vi "Can_File_be_Editted.vi"(0 "Filename":path) -> (1 "File Permissions OK?":bool, 2 "File Status":T1=enum."Directory structure cannot be created", 3 "Comment String":string="Directory structure cannot be created", 4 "Cannot create directory":path)   [LabVIEW 2016]
uses:
  File_Status.ctl
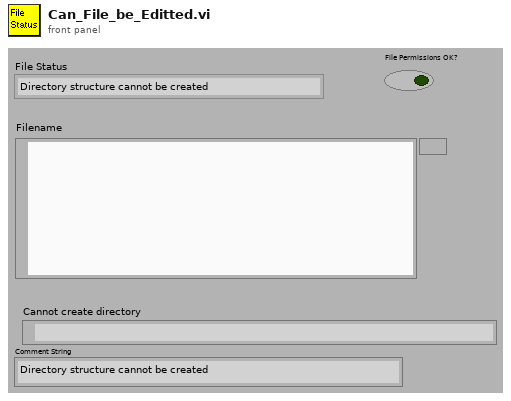
[diagram p1: front panel]
types:
  T1 = typedef "File_Status.ctl" = enum16{"Invalid Path", "File Does not Exist", "This is a folder pathname", "Generic File Error", "Directory structure cannot be created", "File cannot be created", "File can be created", "File exist but read only", "File exist but no access", "File exist with read and write access"}
  T2 = enum16{"read/write", "read-only", "write-only", "write-only (truncate)"}
  T3 = enum16{"open", "replace", "create", "open or create", "replace or create", "replace or create with confirmation"}
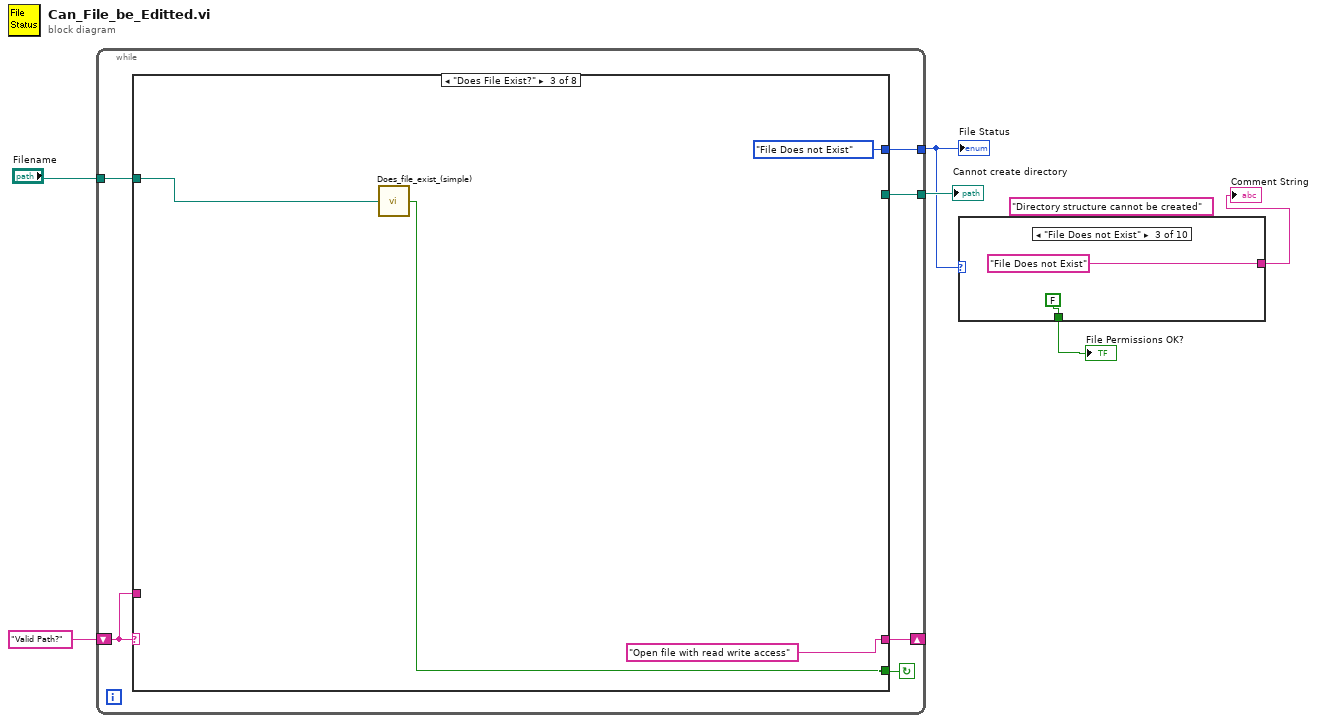
[diagram p0: block diagram]
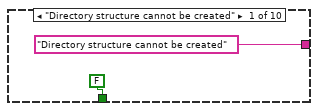
[diagram p2: hidden frame]
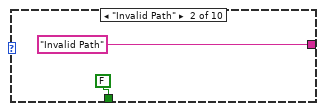
[diagram p3: hidden frame]
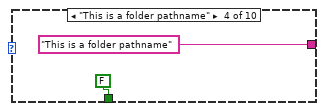
[diagram p4: hidden frame]
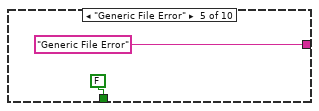
[diagram p5: hidden frame]
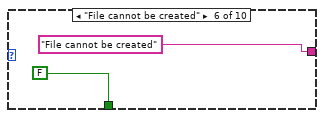
[diagram p6: hidden frame]
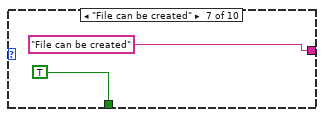
[diagram p7: hidden frame]
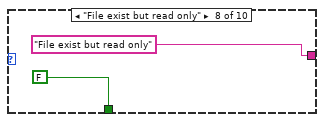
[diagram p8: hidden frame]
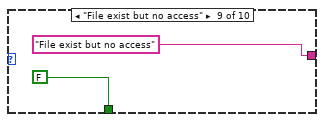
[diagram p9: hidden frame]
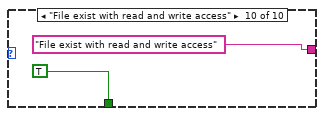
[diagram p10: hidden frame]
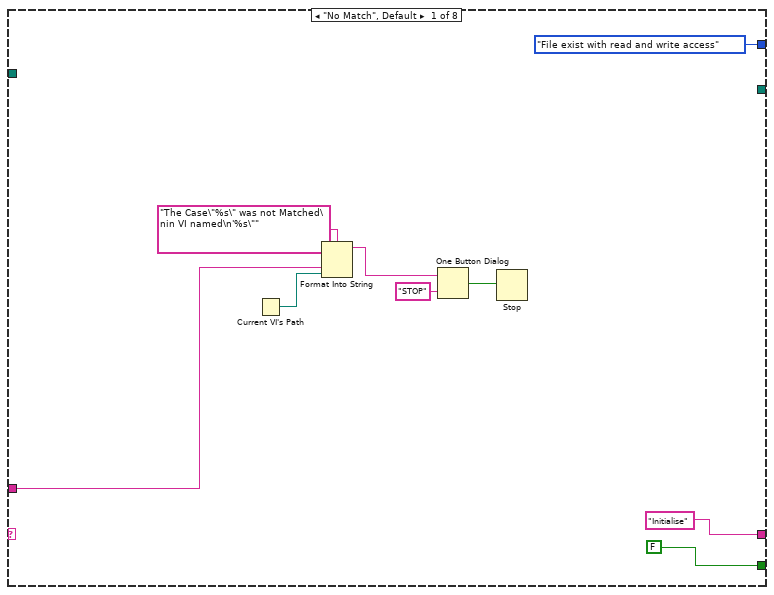
[diagram p11: hidden frame]
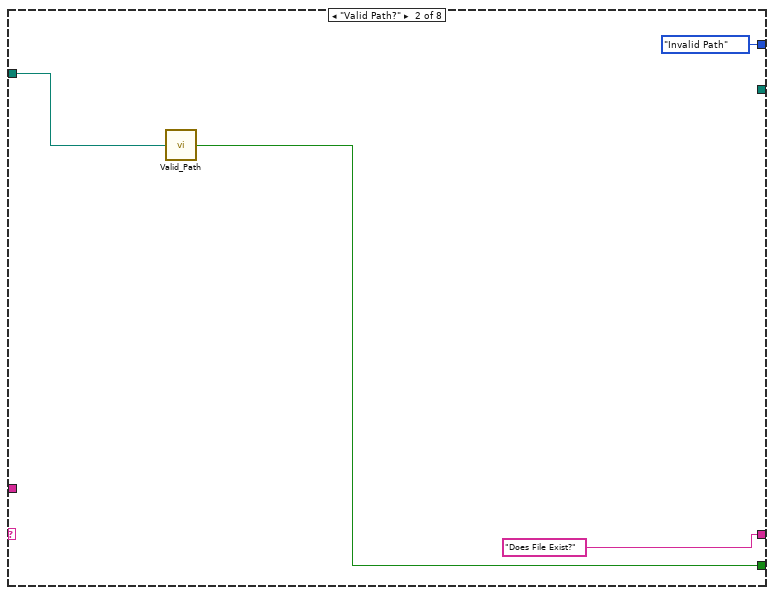
[diagram p12: hidden frame]
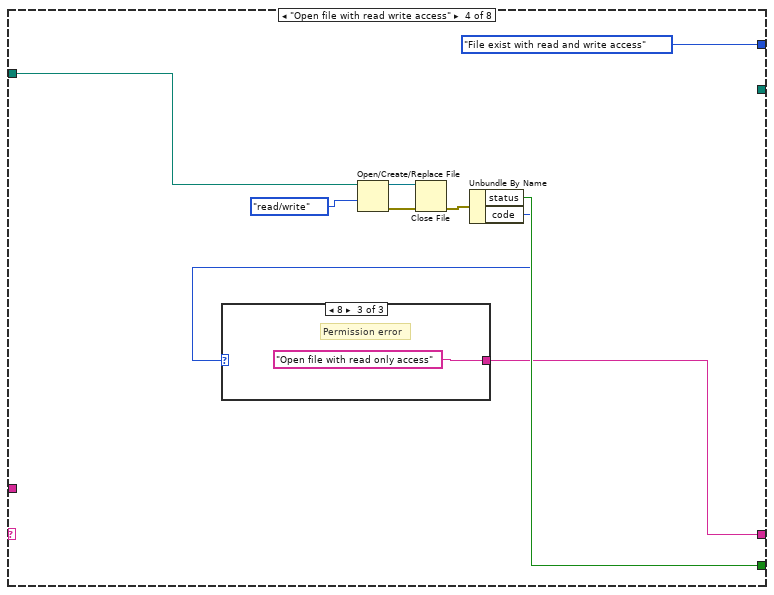
[diagram p13: hidden frame]
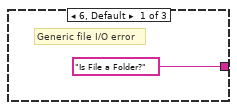
[diagram p14: hidden frame]
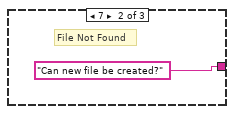
[diagram p15: hidden frame]
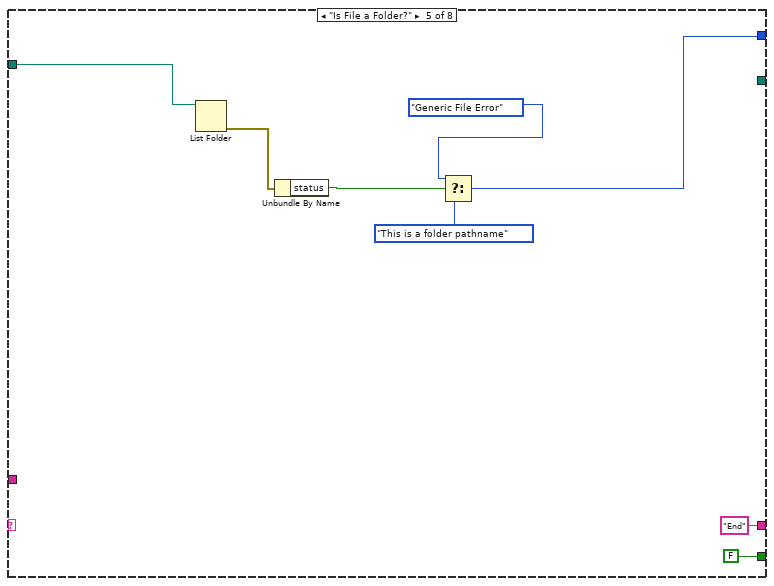
[diagram p16: hidden frame]
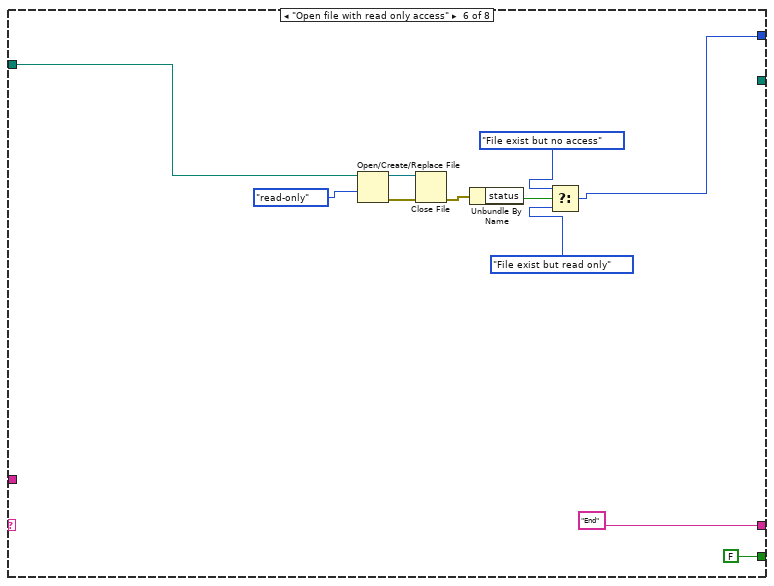
[diagram p17: hidden frame]
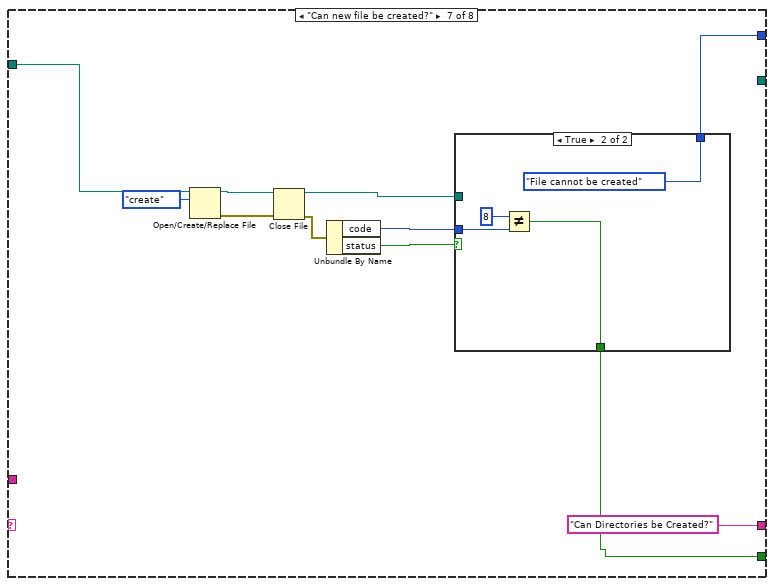
[diagram p18: hidden frame]
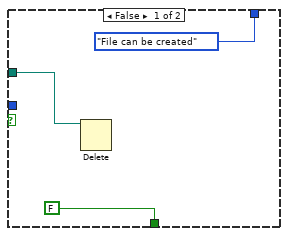
[diagram p19: hidden frame]
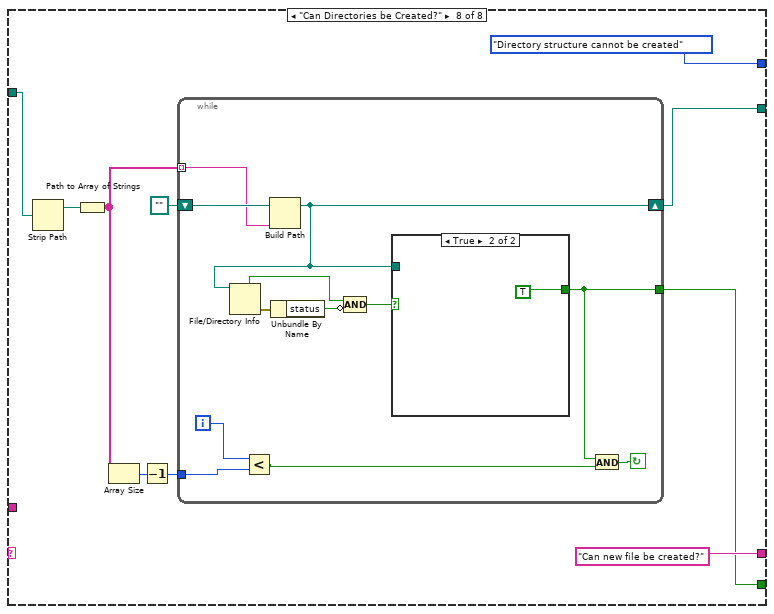
[diagram p20: hidden frame]
diagram:
  (unwired) "Directory structure cannot be created"
  n1 = while {
    shift-left: "Valid Path?" -> [w10]
    shift-right: [w11] -> _
    tunnel: "Filename" -> [w9]
    tunnel: [w8] -> w4
    tunnel: [w7] -> w5
    stop <- w12 continue-if-true
    n2 = case shown="\"Does File Exist?\"" w10 {
      tunnel: [FALSE w23 w26 w33 FALSE ("status") FALSE ("status") w64 w80] -> w12
      tunnel: ["Initialise" "Does File Exist?" "Open file with read write access" w30 "End" ("f") "End" "Can Directories be Created?" "Can new file be created?"] -> w11
      tunnel: w10 -> [w16 _ _ _ _ _ _ _]
      tunnel: w9 -> [_ w24 w27 w35 w49 w55 w66 w86]
      tunnel: [File_Status."File exist with read and write access" ("File Status") File_Status."Invalid Path" ("File Status") File_Status."File Does not Exist" ("File Status") File_Status."File exist with read and write access" ("File Status") w42 w50 w62 File_Status."Directory structure cannot be created" ("File Status")] -> w8
      tunnel: [_ _ _ _ _ _ _ w79] -> w7
      frame "No Match", Default {
        n3 = Current VI's Path() -> (path=w15:path)
        n4 = Format Into String(format string="The Case\"%s\" was not Matched\nin VI named\n'%s\"" ("Format String"), w16, w15) -> (resulting string=w19:string)  [unwired: 2 in, 1 out]
        n5 = One Button Dialog(message=w19, button name ("OK")="STOP") -> (true=w17:bool)
        n6 = Stop(stop? (T)=w17) -> ()
      }
      frame "Valid Path?" {
        n7 = call "Valid_Path.vi"("Filename"=w24) -> ("Valid Path?"=w23:bool)
      }
      frame "Does File Exist?" {
        n8 = call "Does_file_exist_(simple).vi"("Pathname"=w27) -> ("exists?"=w26:bool)
      }
      frame "Open file with read write access" {
        n9 = Open/Create/Replace File(file path (use dialog)=w35, access (0:read/write)=T2."read/write" ("open mode (0)")) -> (refnum out=w36:refnum<file>, error out=w38:errorcluster)  [unwired: 1 in, 4 out]
        n10 = Close File(refnum=w36, error in=w38) -> (error out=w32:errorcluster)  [unwired: 1 out]
        n11 = Unbundle By Name(w32) -> ("status"=w33:bool, "code"=w31:i32)
        n12 = case shown="8" w31 {
          tunnel: ["Is File a Folder?" ("f") "Can new file be created?" ("f") "Open file with read only access"] -> w30
          frame 6, Default {
            # "Generic file I/O error"
          }
          frame 7 {
            # "File Not Found"
          }
          frame 8 {
            # "Permission error"
          }
        }
      }
      frame "Is File a Folder?" {
        n13 = List Folder(path=w49) -> (error out=w48:errorcluster)  [unwired: 1 in, 5 out]
        n14 = Unbundle By Name(w48) -> ("status"=w45:bool)
        n15 = Select(t=File_Status."Generic File Error" ("File Status"), s=w45, f=File_Status."This is a folder pathname" ("File Status")) -> (s? t:f=w42:T1)
      }
      frame "Open file with read only access" {
        n16 = Open/Create/Replace File(file path (use dialog)=w55, access (0:read/write)=T2."read-only" ("open mode (0)")) -> (refnum out=w56:refnum<file>, error out=w59:errorcluster)  [unwired: 1 in, 4 out]
        n17 = Close File(refnum=w56, error in=w59) -> (error out=w58:errorcluster)  [unwired: 1 out]
        n18 = Unbundle By Name(w58) -> ("status"=w53:bool)
        n19 = Select(t=File_Status."File exist but no access" ("File Status"), s=w53, f=File_Status."File exist but read only" ("File Status")) -> (s? t:f=w50:T1)
      }
      frame "Can new file be created?" {
        n20 = Open/Create/Replace File(file path (use dialog)=w66, operation (0:open)=T3."create") -> (refnum out=w70:refnum<file>, error out=w69:errorcluster)  [unwired: 1 in, 4 out]
        n21 = Close File(refnum=w70, error in=w69) -> (path=w65:path, error out=w68:errorcluster)
        n22 = Unbundle By Name(w68) -> ("code"=w63:i32, "status"=w67:bool)
        n23 = case shown="True" w67 {
          tunnel: w65 -> [w74 _]
          tunnel: [FALSE w75] -> w64
          tunnel: w63 -> [_ w78]
          tunnel: [File_Status."File can be created" ("File Status") File_Status."File cannot be created" ("File Status")] -> w62
          frame False {
            n24 = Delete(path (use dialog)=w74) -> ()  [unwired: 1 in, 6 out]
          }
          frame True {
            n25 = Not Equal?(x=8, y=w78) -> (x != y?=w75:bool)
          }
        }
      }
      frame "Can Directories be Created?" {
        n26 = Strip Path(path=w86) -> (stripped path=w81:path)  [unwired: 1 out]
        n27 = Path to Array of Strings(0:w81) -> (2:w83:string[])  [unwired: 1 out]
        n28 = Array Size(array=w83) -> (size(s)=w85:i32)
        n29 = Decrement(x=w85) -> (x-1=w84:i32)
        n30 = while {
          tunnel: [w95] -> w80
          tunnel: w84 -> [w98]
          shift-left: path "" ("appended path") -> [w100]
          shift-right: [w94] -> w79
          tunnel: w83 -> [w99] mode=indexing
          i -> [w89]
          stop <- w96 continue-if-true
          n31 = Less?(x=w89, y=w98) -> (x < y?=w97:bool)
          n32 = Build Path(base path=w100, name or relative path=w99) -> (appended path=w94:path)
          n33 = File/Directory Info(path=w94) -> (directory=w91:bool, error out=w93:errorcluster)  [unwired: 1 in, 5 out]
          n34 = Unbundle By Name(w93) -> ("status"=w92:bool)
          n35 = Compound Arithmetic op=AND(w91, invert w92) -> (w90:bool)
          n36 = case shown="True" w90 {
            tunnel: w94 -> [w104 _]
            tunnel: [w101 TRUE] -> w95
            frame False {
              n37 = Create Folder(path (use dialog)=w104) -> (error out=w103:errorcluster)  [unwired: 1 in, 3 out]
              n38 = Unbundle By Name(w103) -> ("status"=w102:bool)
              n39 = Not(x=w102) -> (.not. x?=w101:bool)
            }
            frame True {
            }
          }
          n40 = And(x=w95, y=w97) -> (x .and. y?=w96:bool)
        }
      }
    }
  }
  "File Status" <- w4
  "Cannot create directory" <- w5
  n41 = case shown="\"File Does not Exist\"" w4 {
    tunnel: [FALSE FALSE FALSE FALSE FALSE FALSE TRUE FALSE FALSE TRUE] -> w3
    tunnel: ["Directory structure cannot be created" "Invalid Path" "File Does not Exist" "This is a folder pathname" "Generic File Error" "File cannot be created" "File can be created" "File exist but read only" "File exist but no access" "File exist with read and write access"] -> w2
    frame "Directory structure cannot be created" {
    }
    frame "Invalid Path" {
    }
    frame "File Does not Exist" {
    }
    frame "This is a folder pathname" {
    }
    frame "Generic File Error" {
    }
    frame "File cannot be created" {
    }
    frame "File can be created" {
    }
    frame "File exist but read only" {
    }
    frame "File exist but no access" {
    }
    frame "File exist with read and write access" {
    }
  }
  "File Permissions OK?" <- w3
  "Comment String" <- w2
